vi "example.vi"   [LabVIEW 2019]
uses:
  mmW_commands/replies/reply_statuscode.ctl
  mmW_commands/mmW_commands.lvlib
types:
  T1 = typedef "mmW_commands.lvlib/reply_statuscode.ctl" = enum16{"Error", "OK"}
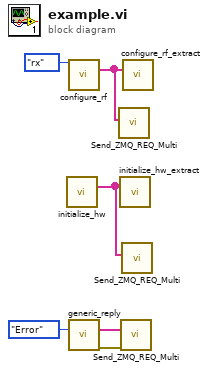
[diagram p0: block diagram]
diagram:
  n1 = call "initialize_hw.vi"() -> ("multipart message"=w4:string[])  [unwired: 13 in, 2 out]
  n2 = call "configure_rf.vi"("port"=enum16{"rx", "tx"}."rx") -> ("multipart message"=w6:string[])  [unwired: 12 in, 2 out]
  n3 = call "generic_reply.vi"("Status (Error)"=reply_statuscode."Error") -> ("multipart message"=w1:string[], "error out"=w2:errorcluster)  [unwired: 12 in, 1 out]
  n4 = call "Send_ZMQ_REQ_Multi.vi"("Data in"=w6) -> ()  [unwired: 8 in, 3 out]
  n5 = call "initialize_hw_extract.vi"("multipart message in"=w4) -> ()  [unwired: 11 in, 4 out]
  n6 = call "Send_ZMQ_REQ_Multi.vi"("error in"=w2, "Data in"=w1) -> ()  [unwired: 7 in, 3 out]
  n7 = call "Send_ZMQ_REQ_Multi.vi"("Data in"=w4) -> ()  [unwired: 8 in, 3 out]
  n8 = call "configure_rf_extract.vi"("multipart message in"=w6) -> ()  [unwired: 9 in, 6 out]
